vi "pmu_Phasors Block (Std 2011).vi"(6 "init meas data":u8[](array[numeric]), 8 "measurement data":T1 {"data error" format="%02b"; "PMU time quality" format="%03b"; "time quality" format="%08b"; "trigger reason" format="%04b"}, 9 "data format":u16, 10 "phasor units":u32[](array[numeric]), 11 "nominal frequency":enum16{"50 Hz", "60 Hz"}(ring)) -> (0 "df/dt out of range":bool, 1 "freq out of range":bool, 2 "phasor out of range":bool, 3 "data block":u8[](array[numeric]) format="%b", 4 "analog out of range":bool)   [LabVIEW 2013, in "NI_EP_PMU.lvlib"]
doc: "This VI converts phasor data cluster to binary data block."
uses:
  <vilib>/addons/Electrical Power/PMU/NI_EP_PMU.lvlib
  <vilib>/addons/Electrical Power/PMU/Common/Controls/pmu_Measurement Data (Std 2011).ctl
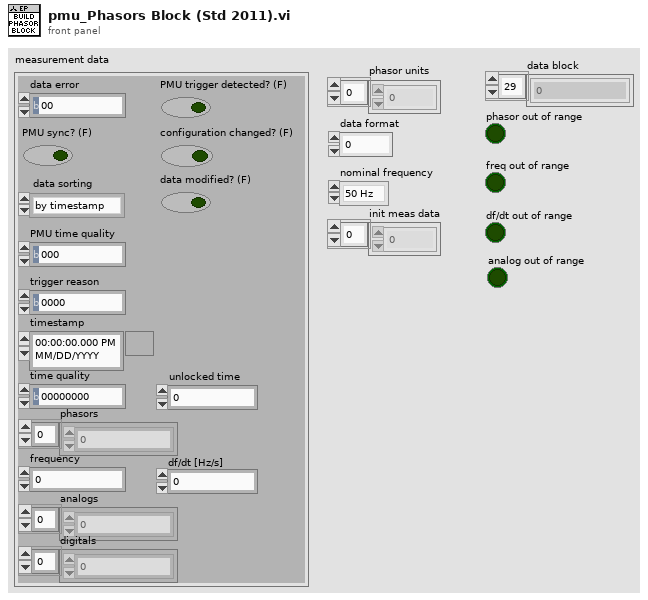
[diagram p1: front panel]
types:
  T1 = typedef "NI_EP_PMU.lvlib/pmu_Measurement Data (Std 2011).ctl" = cluster{"data error":u8, "PMU sync? (F)":bool, "data sorting":enum16{"by timestamp", "by arrival"}, "PMU trigger detected? (F)":bool, "configuration changed? (F)":bool, "data modified? (F)":bool, "PMU time quality":u8, "unlocked time":u32, "trigger reason":u8, "df/dt [Hz/s]":sgl, "analogs":sgl[], "digitals":u16[], "frequency":sgl, "phasors":csg[], "timestamp":timestamp, "time quality":u8}
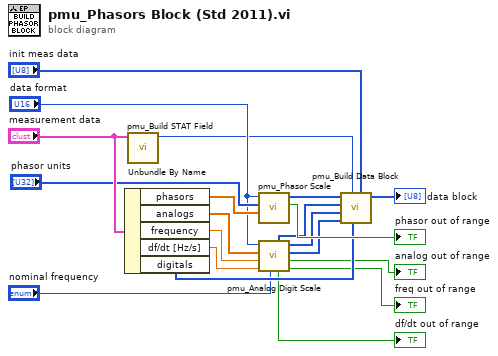
[diagram p0: block diagram]
diagram:
  n1 = Unbundle By Name("measurement data") -> ("phasors"=w14:csg[], "analogs"=w12:sgl[], "frequency"=w11:sgl, "df/dt [Hz/s]"=w10:sgl, "digitals"=w9:u16[])
  n2 = call <vilib>:"pmu_Build STAT Field.vi"("measurement data"="measurement data") -> ("STAT field"=w5:u16)  [unwired: 10 in]
  n3 = call <vilib>:"pmu_Phasor Scale.vi"("phasors in"=w14, "phasor units"="phasor units", "format"="data format") -> ("phasor out of range"=→"phasor out of range":bool, "phasor byte array"=w17:u8[])  [unwired: 7 in]
  n4 = call <vilib>:"pmu_Analog Digit Scale.vi"("nominal frequency"="nominal frequency", "dfreq in"=w10, "freq in"=w11, "analogs in"=w12, "format"="data format") -> ("freq out of range"=→"freq out of range":bool, "analog out of range"=→"analog out of range":bool, "analogs byte array"=w6:u8[], "dfreq byte array"=w7:u8[], "df/dt out of range"=→"df/dt out of range":bool, "freq byte array"=w8:u8[])  [unwired: 1 in]
  n5 = call <vilib>:"pmu_Build Data Block.vi"("init meas data"="init meas data", "digitals"=w9, "STAT field"=w5, "analogs byte array"=w6, "dfreq byte array"=w7, "freq byte array"=w8, "phasor byte array"=w17) -> ("data block"=→"data block":u8[])  [unwired: 4 in]
